vi "ButterworthBandCalculator.vi"(6 "Settling":enum16{"99%", "99,9%"}(ring)=enum."99,9%", 8 "Filter Order":u32=1 min=1 max=4, 10 "Regime time":dbl=0.1, 11 "ADC Sample Rate":dbl=50000000.0) -> (0 "Single stage freq. [Hz]":dbl, 1 "Time constant [s]":dbl, 2 "N. stages":u32, 3 "IIR Filter out":T1 {"Forward Coefficients" format="%.4f"; "Reverse Coefficients" format="%.4f"}, 4 "Effective freq. [Hz]":dbl)   [LabVIEW 2019, in "FPGA.lvlib"]
uses:
  FPGA.lvlib
  <vilib>/Analysis/3filter.llb/Filter Passband Type.ctl
  <vilib>/Analysis/NI_AALBase.lvlib
panel:
  out "Sampling freq. [Hz]":dbl
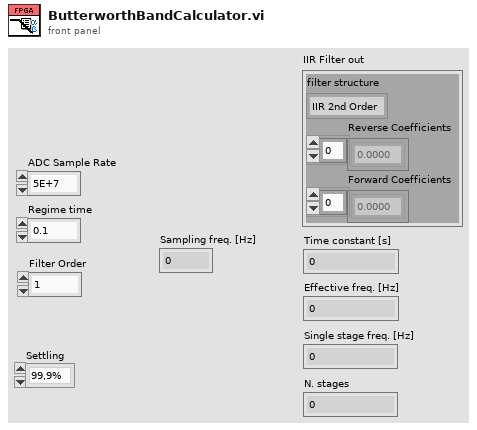
[diagram p1: front panel]
types:
  T1 = cluster{"filter structure":enum32{"IIR 2nd Order", "IIR 4th Order"}, "Reverse Coefficients":dbl[], "Forward Coefficients":dbl[]}
  T2 = typedef "NI_AALBase.lvlib/Filter Passband Type.ctl" = enum32{"Lowpass", "Highpass", "Bandpass", "Bandstop"}
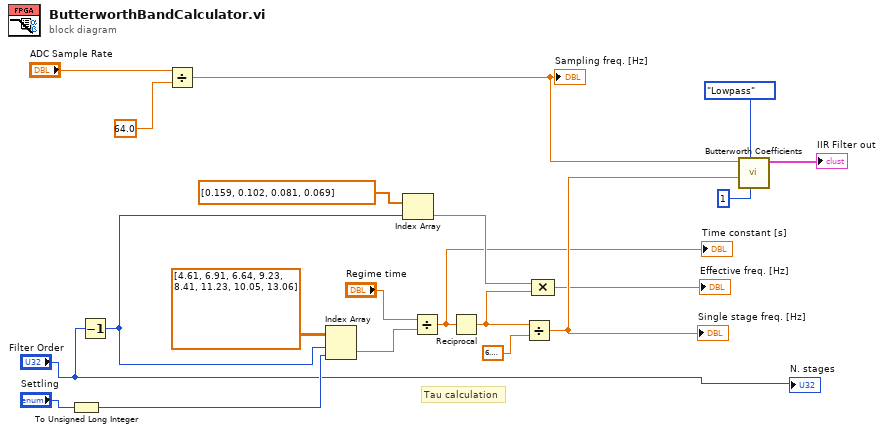
[diagram p0: block diagram]
diagram:
  # "Tau calculation"
  n1 = To Unsigned Long Integer(number="Settling") -> (unsigned 32bit integer=w3:u32)
  n2 = Decrement(x="Filter Order") -> (x-1=w1:u32)
  n3 = Divide(x="ADC Sample Rate", y=64.0) -> (x/y=w12:dbl)
  "Sampling freq. [Hz]" <- w12
  n4 = Index Array(array=dbl[][] [[4.61, 6.91], [6.64, 9.23], [8.41, 11.23], [10.05, 13.06]], index (row)=w1, index (col)=w3) -> (element=w18:dbl)
  n5 = Index Array(array=dbl[] [0.159, 0.102, 0.081, 0.069], index=w1) -> (element=w16:dbl)
  n6 = Divide(x="Regime time", y=w18) -> (x/y=w5:dbl)
  "Time constant [s]" <- w5
  n7 = Reciprocal(x=w5) -> (1/x=w9:dbl)
  n8 = Divide(x=w9, y=6.283185307179586) -> (x/y=w8:dbl)
  "Single stage freq. [Hz]" <- w8
  n9 = Compound Arithmetic op=MULTIPLY(w16, w9) -> (→"Effective freq. [Hz]":dbl)
  n10 = call <vilib>:"Butterworth Coefficients.vi"("order"=1, "filter type"=Filter_Passband_Type."Lowpass", "low cutoff freq: fl"=w8, "sampling freq: fs"=w12) -> ("IIR Filter Cluster"=→"IIR Filter out":T1)  [unwired: 6 in, 1 out]
  "N. stages" <- "Filter Order"
